vi "ThermocoupleRead.vi"(0 "Array in":dbl[](array[numeric]), 1 "Numeric 8":dbl, 2 "Numeric 9":dbl, 3 "Numeric 3":dbl, 5 "Numeric 2":dbl, 7 "Numeric 4":dbl, 9 "Numeric 5":dbl, 11 "Numeric 6":dbl, 12 "Numeric 7":dbl, 13 "Numeric 10":dbl, 14 "Numeric 11":dbl) -> (4 "Array out":dbl[](array[numeric]))   [LabVIEW 2017]
uses:
  <vilib>/ptbypt/NI_PtbyPt.lvlib
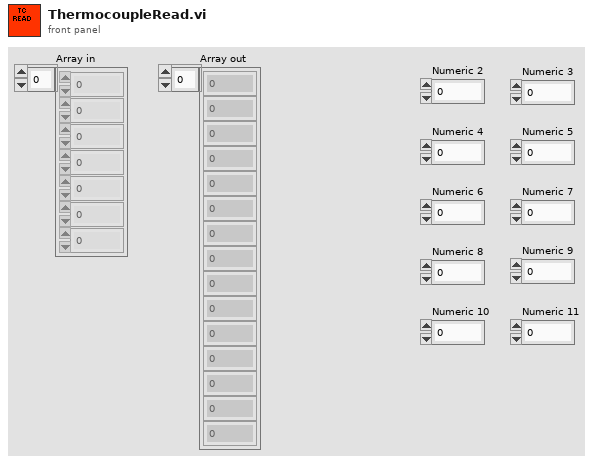
[diagram p1: front panel]
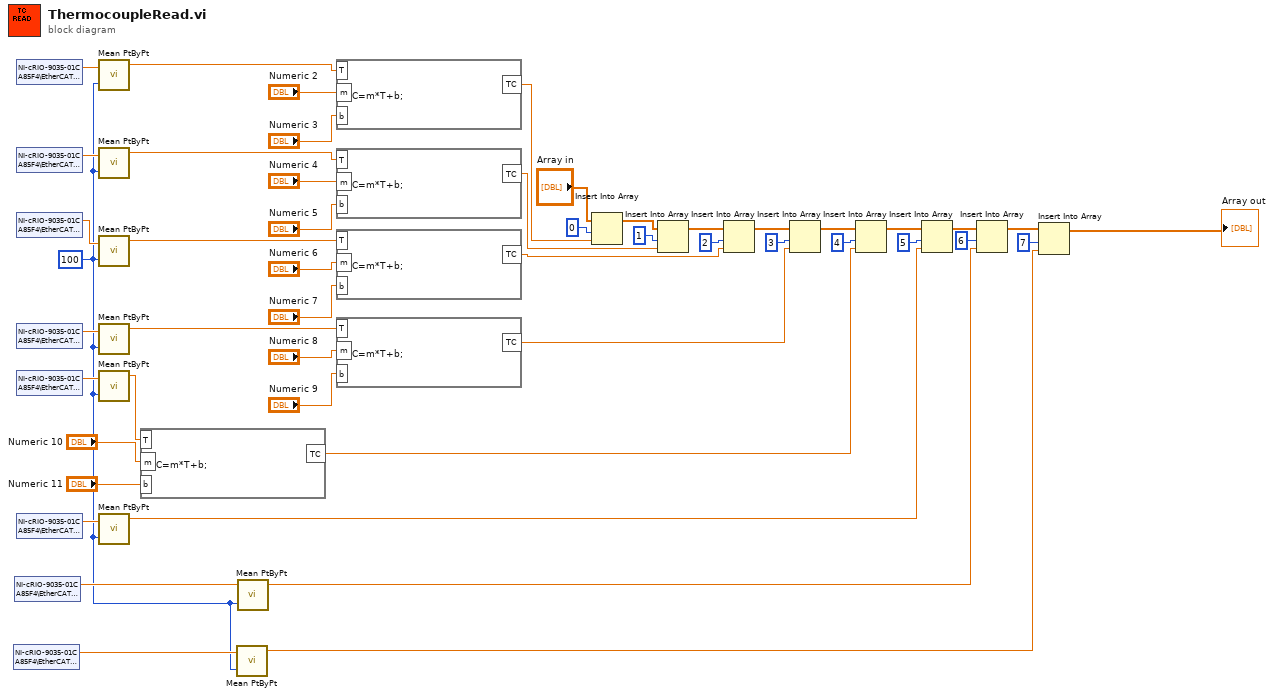
[diagram p0: block diagram]
diagram:
  w1 = 100
  n1 = shared-variable "NI-cRIO-9035-01CA85F4\\EtherCAT Master\\Device\\Mod2\\TC7"() -> (w3:dbl)  [unwired: 1 in, 1 out]
  n2 = shared-variable "NI-cRIO-9035-01CA85F4\\EtherCAT Master\\Device\\Mod2\\TC6"() -> (w5:dbl)  [unwired: 1 in, 1 out]
  n3 = shared-variable "NI-cRIO-9035-01CA85F4\\EtherCAT Master\\Device\\Mod2\\TC0"() -> (w42:dbl)  [unwired: 1 in, 1 out]
  n4 = shared-variable "NI-cRIO-9035-01CA85F4\\EtherCAT Master\\Device\\Mod2\\TC1"() -> (w43:dbl)  [unwired: 1 in, 1 out]
  n5 = shared-variable "NI-cRIO-9035-01CA85F4\\EtherCAT Master\\Device\\Mod2\\TC2"() -> (w44:dbl)  [unwired: 1 in, 1 out]
  n6 = shared-variable "NI-cRIO-9035-01CA85F4\\EtherCAT Master\\Device\\Mod2\\TC3"() -> (w45:dbl)  [unwired: 1 in, 1 out]
  n7 = shared-variable "NI-cRIO-9035-01CA85F4\\EtherCAT Master\\Device\\Mod2\\TC4"() -> (w36:dbl)  [unwired: 1 in, 1 out]
  n8 = shared-variable "NI-cRIO-9035-01CA85F4\\EtherCAT Master\\Device\\Mod2\\TC5"() -> (w12:dbl)  [unwired: 1 in, 1 out]
  n9 = call <vilib>:"Mean PtByPt.vi"("x"=w42, "sample length"=w1) -> ("mean"=w34:dbl)  [unwired: 2 in, 1 out]
  n10 = call <vilib>:"Mean PtByPt.vi"("x"=w43, "sample length"=w1) -> ("mean"=w32:dbl)  [unwired: 2 in, 1 out]
  n11 = call <vilib>:"Mean PtByPt.vi"("x"=w44, "sample length"=w1) -> ("mean"=w30:dbl)  [unwired: 2 in, 1 out]
  n12 = call <vilib>:"Mean PtByPt.vi"("x"=w45, "sample length"=w1) -> ("mean"=w22:dbl)  [unwired: 2 in, 1 out]
  n13 = call <vilib>:"Mean PtByPt.vi"("x"=w36, "sample length"=w1) -> ("mean"=w16:dbl)  [unwired: 2 in, 1 out]
  n14 = call <vilib>:"Mean PtByPt.vi"("x"=w12, "sample length"=w1) -> ("mean"=w11:dbl)  [unwired: 2 in, 1 out]
  n15 = formula code="TC=m*T+b;"("T"=w16, "m"="Numeric 10", "b"="Numeric 11") -> ("TC"=w15:dbl)
  n16 = call <vilib>:"Mean PtByPt.vi"("x"=w3, "sample length"=w1) -> ("mean"=w2:dbl)  [unwired: 2 in, 1 out]
  n17 = call <vilib>:"Mean PtByPt.vi"("x"=w5, "sample length"=w1) -> ("mean"=w4:dbl)  [unwired: 2 in, 1 out]
  n18 = formula code="TC=m*T+b;"("T"=w34, "m"="Numeric 2", "b"="Numeric 3") -> ("TC"=w33:dbl)
  n19 = formula code="TC=m*T+b;"("T"=w32, "m"="Numeric 4", "b"="Numeric 5") -> ("TC"=w31:dbl)
  n20 = formula code="TC=m*T+b;"("T"=w30, "m"="Numeric 6", "b"="Numeric 7") -> ("TC"=w29:dbl)
  n21 = formula code="TC=m*T+b;"("T"=w22, "m"="Numeric 8", "b"="Numeric 9") -> ("TC"=w19:dbl)
  n22 = Insert Into Array(array="Array in", index=0, new element=w33) -> (w40:dbl[])
  n23 = Insert Into Array(array=w40, index=1, new element=w31) -> (w46:dbl[])
  n24 = Insert Into Array(array=w46, index=2, new element=w29) -> (w47:dbl[])
  n25 = Insert Into Array(array=w47, index=3, new element=w19) -> (w37:dbl[])
  n26 = Insert Into Array(array=w37, index=4, new element=w15) -> (w14:dbl[])
  n27 = Insert Into Array(array=w14, index=5, new element=w11) -> (w8:dbl[])
  n28 = Insert Into Array(array=w8, index=6, new element=w4) -> (w7:dbl[])
  n29 = Insert Into Array(array=w7, index=7, new element=w2) -> (→"Array out":dbl[])
